vi "Get Parameters (SubVI).vi"(5 "Command":string="?", 8 "error in (no error)":errorcluster, 11 "VISA Refnum in":refnum<visa-resource-name>) -> (0 "error out":errorcluster, 1 "Array":string[](array[string]), 2 "Response":string, 3 "VISA Refnum out":refnum<visa-resource-name>)   [LabVIEW 2015]
uses:
  Library/Token.ctl
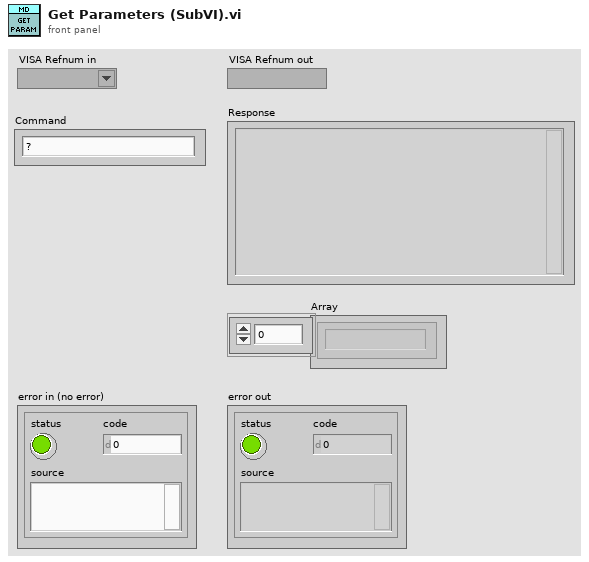
[diagram p1: front panel]
types:
  T1 = typedef "Token.ctl" = enum16{"End", "Boolean", "Named Cluster", "Unnamed Cluster", "Array", "String", "Decimal", "FloatingPoint", "End Array", "End Cluster"}
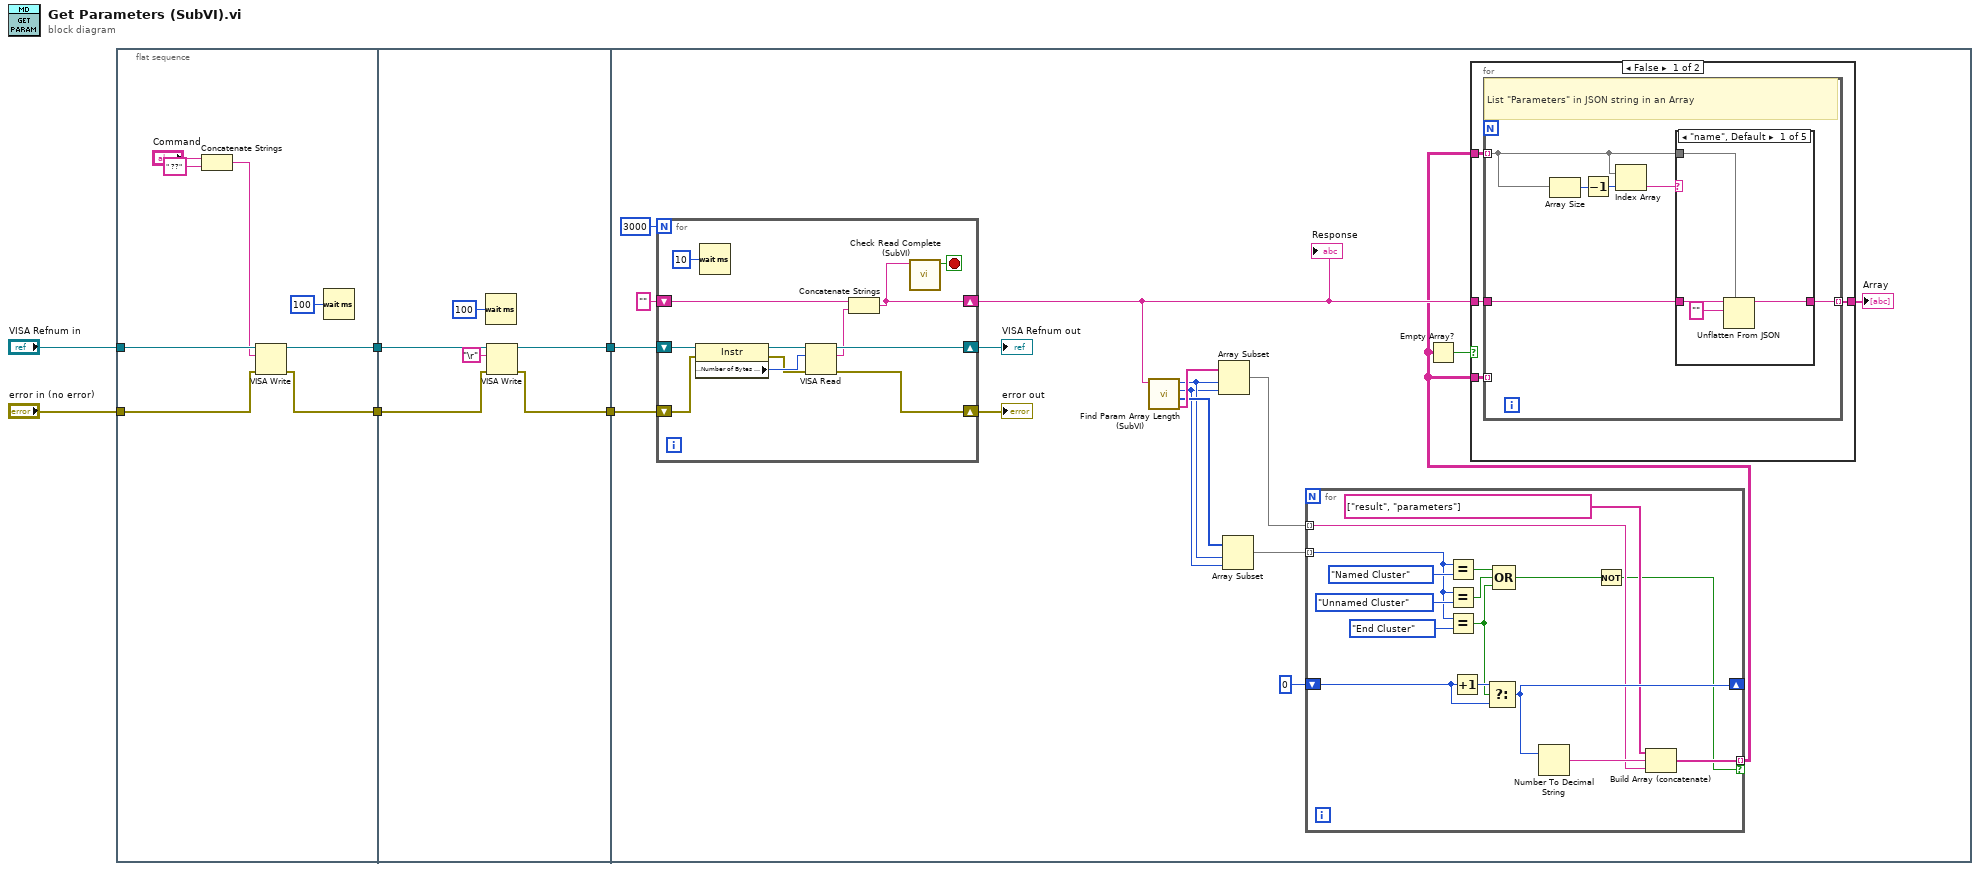
[diagram p0: block diagram]
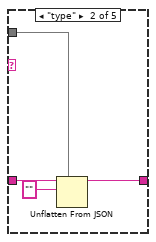
[diagram p2: hidden frame]
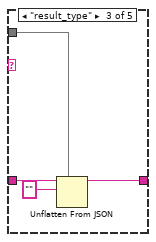
[diagram p3: hidden frame]
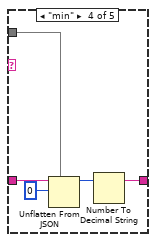
[diagram p4: hidden frame]
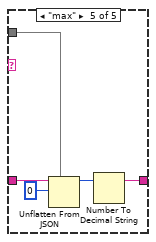
[diagram p5: hidden frame]
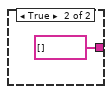
[diagram p6: hidden frame]
diagram:
  n1 = flat-sequence {
    tunnel: "VISA Refnum in" -> [w12]
    tunnel: "error in (no error)" -> [w10]
    tunnel: [w9] -> w6
    tunnel: [w11] -> w5
    tunnel: [w15] -> w4
    tunnel: [w17] -> w3
    tunnel: w6 -> [w16]
    tunnel: w5 -> [w18]
    tunnel: w4 -> [w36]
    tunnel: w3 -> [w35]
    frame #0 {
      n2 = Concatenate Strings("Command", " ??" ("string")) -> (w8:string)
      n3 = VISA Write(VISA resource name=w12, write buffer=w8, error in (no error)=w10) -> (VISA resource name out=w11:refnum<visa-resource-name>, error out=w9:errorcluster)  [unwired: 1 out]
      n4 = Wait (ms)(milliseconds to wait=u32 100) -> ()  [unwired: 1 out]
    }
    frame #1 {
      n5 = Wait (ms)(milliseconds to wait=u32 100) -> ()  [unwired: 1 out]
      n6 = VISA Write(VISA resource name=w18, write buffer="\r", error in (no error)=w16) -> (VISA resource name out=w17:refnum<visa-resource-name>, error out=w15:errorcluster)  [unwired: 1 out]
    }
    frame #2 {
      n7 = for {
        N: 3000 -> [_]
        shift-right: [w98] -> w33
        shift-left: w35 -> [w96]
        shift-right: [w97] -> w34
        shift-left: w36 -> [w90]
        shift-right: [w87] -> w30
        shift-left: "" -> [w92]
        stop <- w88 stop-if-true
        n8 = property class="Instr"(reference=w96, error in=w90) -> (reference out=w94:refnum<visa-resource-name>, error out=w89:errorcluster, "Serial Settings:Number of Bytes at Serial Port"=w93:u32)
        n9 = Wait (ms)(milliseconds to wait=u32 10) -> ()  [unwired: 1 out]
        n10 = VISA Read(VISA resource name=w94, byte count=w93, error in (no error)=w89) -> (VISA resource name out=w98:refnum<visa-resource-name>, read buffer=w95:string, error out=w97:errorcluster)  [unwired: 1 out]
        n11 = Concatenate Strings(w92, w95) -> (w87:string)
        n12 = call "Check Read Complete (SubVI).vi"("JSON String"=w87) -> ("Complete?"=w88:bool)  [unwired: 10 in]
      }
      "error out" <- w34
      "VISA Refnum out" <- w33
      "Response" <- w30
      n13 = call "Find Param Array Length (SubVI).vi"("JSON String"=w30) -> ("Variable Array"=w28:string[], "Token Array"=w27:T1[], "Length"=w25:i32, "Index"=w26:i32)  [unwired: 7 in]
      n14 = Array Subset(array=w28, index=w26, length=w25) -> (w22:string[])
      n15 = Array Subset(array=w27, index=w26, length=w25) -> (w24:T1[])
      n16 = for {
        tunnel: w24 -> [w48] mode=indexing
        shift-right: [w44] -> _
        shift-left: 0 -> [w52]
        tunnel: w22 -> [w42] mode=indexing
        tunnel: [w40] -> w21 mode=indexing if=w38
        n17 = Equal?(x=w48, y=Token."Named Cluster") -> (x = y?=w47:bool)
        n18 = Equal?(x=w48, y=Token."Unnamed Cluster") -> (x = y?=w46:bool)
        n19 = Equal?(x=w48, y=Token."End Cluster") -> (x = y?=w45:bool)
        n20 = Increment(x=w52) -> (x+1=w53:i32)
        n21 = Select(t=w53, s=w45, f=w52) -> (s? t:f=w44:i32)
        n22 = Compound Arithmetic op=OR(w47, w46, w45) -> (w39:bool)
        n23 = Number To Decimal String(number=w44) -> (decimal integer string=w43:string)  [unwired: 1 in]
        n24 = Not(x=w39) -> (.not. x?=w38:bool)
        n25 = Build Array (concatenate)(string[] ["result", "parameters"], w43, w42) -> (w40:string[])
      }
      n26 = Empty Array?(array=w21) -> (empty?=w29:bool)
      n27 = case shown="False" w29 {
        tunnel: [w57 string[] []] -> w37
        tunnel: w21 -> [w56 _]
        tunnel: w30 -> [w55 _]
        tunnel: w21 -> [w54 _]
        frame False {
          n28 = for {
            tunnel: w55 -> [w63]
            tunnel: [w62] -> w57 mode=indexing
            tunnel: w56 -> [w58] mode=indexing
            tunnel: w54 -> [_] mode=indexing
            # "List \"Parameters\" in JSON string in an Array"
            n29 = Array Size(array=w58) -> (size(s)=w61:i32)
            n30 = Decrement(x=w61) -> (x-1=w60:i32)
            n31 = Index Array(array=w58, index=w60) -> (element=w59:string)
            n32 = case shown="\"name\", Default" w59 {
              tunnel: w63 -> [w67 w71 w75 w80 w85]
              tunnel: [w65 w69 w73 w76 w81] -> w62
              tunnel: w58 -> [w64 w68 w72 w78 w83]
              frame "name", Default {
                n33 = Unflatten From JSON(path=w64, JSON string=w67, type and defaults="" ("JSON string")) -> (value=w65:string)  [unwired: 4 in, 1 out]
              }
              frame "type" {
                n34 = Unflatten From JSON(path=w68, JSON string=w71, type and defaults="" ("JSON string")) -> (value=w69:string)  [unwired: 4 in, 1 out]
              }
              frame "result_type" {
                n35 = Unflatten From JSON(path=w72, JSON string=w75, type and defaults="" ("JSON string")) -> (value=w73:string)  [unwired: 4 in, 1 out]
              }
              frame "min" {
                n36 = Unflatten From JSON(path=w78, JSON string=w80, type and defaults=0) -> (value=w79:i32)  [unwired: 4 in, 1 out]
                n37 = Number To Decimal String(number=w79) -> (decimal integer string=w76:string)  [unwired: 1 in]
              }
              frame "max" {
                n38 = Unflatten From JSON(path=w83, JSON string=w85, type and defaults=0) -> (value=w84:i32)  [unwired: 4 in, 1 out]
                n39 = Number To Decimal String(number=w84) -> (decimal integer string=w81:string)  [unwired: 1 in]
              }
            }
          }
        }
        frame True {
        }
      }
      "Array" <- w37
    }
  }
